vi "PathPlanner_GoalEndState_New.vi"(9 "Rotation":T1={"VALUE"=0.0, "COS"=1.0, "SIN"=0.0} {"SIN" format="%13.4f"; "COS" format="%13.4f"; "VALUE" format="%13.4f"}, 11 "Velocity":dbl) -> (3 "GoalEndState":T2={"Velocity"=0.0, "Rotation"={"VALUE"=0.0, "COS"=1.0, "SIN"=0.0}} {"Rotation"."SIN" format="%13.4f"; "Rotation"."COS" format="%13.4f"; "Rotation"."VALUE" format="%13.4f"})   [LabVIEW 2019, in "PathPlanner.lvlib"]
doc: "Describes the goal end state of the robot when finishing a path */\n\nCreate a new goal end state\n\nInputs: \n -- velocity - double - The goal end velocity (M/S)\n -- rotation - rotation2d - The goal rotation\n\nOutputs:\n -- GoalEndState - cluster - data structure"
uses:
  PathPlanner.lvlib
  TypeDef/PathPlannerGoalEndState.ctl
  <vilib>/Rock Robotics/WPI/ThirdParty/JAS_Junk/TrajLib/TypeDef/ROTATION2D.ctl
  <vilib>/Rock Robotics/WPI/ThirdParty/JAS_Junk/TrajLib/Trajectory_Library.lvlib
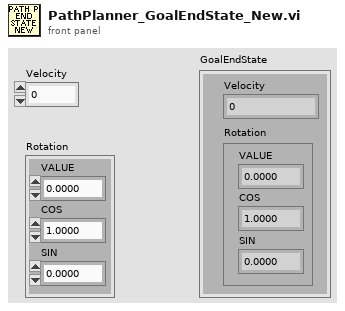
[diagram p1: front panel]
types:
  T1 = typedef "Trajectory_Library.lvlib/ROTATION2D.ctl" = cluster{"VALUE":dbl, "COS":dbl, "SIN":dbl}
  T2 = typedef "PathPlanner.lvlib/PathPlannerGoalEndState.ctl" = cluster{"Velocity":dbl, "Rotation":T1}
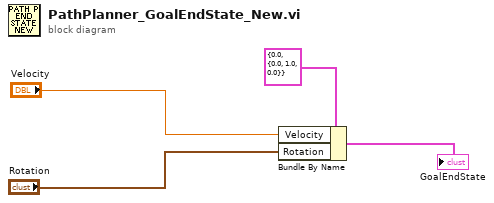
[diagram p0: block diagram]
diagram:
  n1 = Bundle By Name(cluster=T2 {"Velocity"=0.0, "Rotation"={"VALUE"=0.0, "COS"=1.0, "SIN"=0.0}} ("GoalEndState"), "Velocity"="Velocity", "Rotation"="Rotation") -> (→"GoalEndState":T2)
